vi "Teleop.vi"(10 "Match Info":T1={"Autonomous Elapsed Seconds"=0.0, "TeleOp Elapsed Seconds"=0.0, "Disabled Elapsed Seconds"=0.0, "Visited Autonomous"=FALSE, "Visited TeleOp"=FALSE, "Visited Disabled"=FALSE, "Autonomous Settings"={"Autonomous Style"=enum."Independent", "VI Refnum"=refnum}}, 11 "Call Context":T2) -> ()   [LabVIEW 2015]
doc: "This VI is called for each TeleOp packet received from the DS where the robot is not disabled. It is often used to read from the joysticks and update I/O or to update setpoints for timed control loops. It should complete and return within 20 milliseconds or it may miss DS packets."
uses:
  <vilib>/Rock Robotics/WPI/DriverStation/WPI_DriverStationDerivedRobotMode.ctl
  <vilib>/Rock Robotics/WPI/DriverStation/WPI_DriverStationMatch Info.ctl
  <vilib>/Rock Robotics/WPI/Solenoid/WPI_SolenoidValue.ctl
  <vilib>/Rock Robotics/WPI/Utilities/WPI_GetSetVariantRefNum.vi
  <vilib>/Rock Robotics/Network Tables/NT Write Boolean Array.vi
  <vilib>/Rock Robotics/Network Tables/NT Write Numeric Array.vi
  <vilib>/Rock Robotics/Network Tables/NT Read Boolean.vi
  <vilib>/Rock Robotics/Network Tables/NT Read Number.vi
  <vilib>/Rock Robotics/WPI/Solenoid/WPI_SolenoidSetEnum.vi
panel:
  out "Compressor Running":bool
  out "Enabled":bool
  out "Sample Slider 0":dbl(slide) scale=0.0..5.0
  out "Sample Boolean 1":bool
  out "Sample Boolean 0":bool
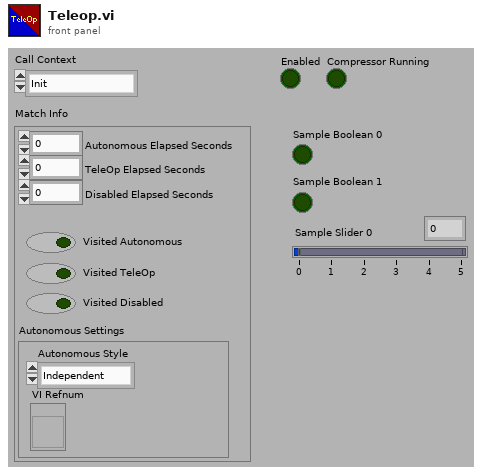
[diagram p1: front panel]
types:
  T1 = typedef "WPI_DriverStationMatch Info.ctl" = cluster{"Autonomous Elapsed Seconds":dbl, "TeleOp Elapsed Seconds":dbl, "Disabled Elapsed Seconds":dbl, "Visited Autonomous":bool, "Visited TeleOp":bool, "Visited Disabled":bool, "Autonomous Settings":cluster{"Autonomous Style":enum16{"Iterative", "Independent"}, "VI Refnum":refnum<vi>}}
  T2 = typedef "WPI_DriverStationDerivedRobotMode.ctl" = enum16{"Init", "Execute", "Stop"}
  T3 = typedef "WPI_SolenoidValue.ctl" = enum16{"Off", "On", "Forward", "Reverse"}
  T4 = typedef "WPI_RobotDriveDevRef.ctl" = cluster{"DevStatus":errorcluster, "Motors[]":T5[], "Square Inputs":bool, "Max Output":dbl}
  T5 = typedef "WPI_MotorControlDeviceRef.ctl" = cluster{"DeviceStatus":errorcluster, "Type":T6, "PWM":cluster{"PWM Channel":T7, "DeadBand":T8}, "CAN":cluster{"Device Number":u8, "Control Mode":T9, "Semaphore":T10, "Max Vout":dbl, "TalonSRX Control Mode":T11}, "Invert":bool}
  T6 = typedef "WPI_MotorControlType.ctl" = enum16{"PWM", "CAN", "CANTalonSRX"}
  T7 = typedef "FPGA_DIOPWMChannel.ctl" = enum8{"PWM 0", "PWM 1", "PWM 2", "PWM 3", "PWM 4", "PWM 5", "PWM 6", "PWM 7", "PWM 8", "PWM 9", "PWM MXP 0", "PWM MXP 1", "PWM MXP 2", "PWM MXP 3", "PWM MXP 4", "PWM MXP 5", "PWM MXP 6", "PWM MXP 7", "PWM MXP 8", "PWM MXP 9", "Invalid"}
  T8 = typedef "WPI_PWMDeadband.ctl" = cluster{"Name":string, "maxPositivePwm":i32, "minPositivePwm":i32, "centerPwm":i32, "maxNegativePwm":i32, "minNegativePwm":i32, "angularRange":u16}
  T9 = typedef "WPI_CANJaguar_ControlMode.ctl" = enum8{"Percent VBus", "Current", "Speed", "Position", "Voltage"}
  T10 = typedef "Semaphore RefNum" = refnum<k1>
  T11 = typedef "WPI_CANTalonSRX_APIControlMode.ctl" = enum8{"Percent VBus", "Speed", "Position", "Slave", "Unchanged / Invalid", "Voltage Compensation", "Current", "Motion Profile"}
  T12 = typedef "WPI_JoystickDevRef.ctl" = cluster{"Device":T13}
  T13 = typedef "WPI_JoystickDeviceEnum.ctl" = enum16{"USB 0", "USB 1", "USB 2", "USB 3", "USB 4", "USB 5"}
  T14 = typedef "WPI_CompressorDevRef.ctl" = cluster{"DevStatus":errorcluster, "Pneumatics Control Module":u8}
  T15 = typedef "WPI_DigitalInputDevRef.ctl" = cluster{"DevStatus":errorcluster, "DIO Channel":T16}
  T16 = typedef "FPGA_DIOChannel.ctl" = enum8{"DIO 0", "DIO 1", "DIO 2", "DIO 3", "DIO 4", "DIO 5", "DIO 6", "DIO 7", "DIO 8", "DIO 9", "DIO MXP 0", "DIO MXP 1", "DIO MXP 2", "DIO MXP 3", "DIO MXP 4", "DIO MXP 5", "DIO MXP 6", "DIO MXP 7", "DIO MXP 8", "DIO MXP 9", "DIO MXP 10", "DIO MXP 11", "DIO MXP 12", "DIO MXP 13", "DIO MXP 14", "DIO MXP 15", "Invalid"}
  T17 = typedef "WPI_SolenoidDevRef.ctl" = cluster{"DevStatus":errorcluster, "Pneumatics Control Module":u8, "Forward Solenoid Channel":T18, "Reverse Solenoid Channel":T18}
  T18 = typedef "WPI_SolenoidChannel.ctl" = enum8{"Solenoid 0", "Solenoid 1", "Solenoid 2", "Solenoid 3", "Solenoid 4", "Solenoid 5", "Solenoid 6", "Solenoid 7", "Invalid"}
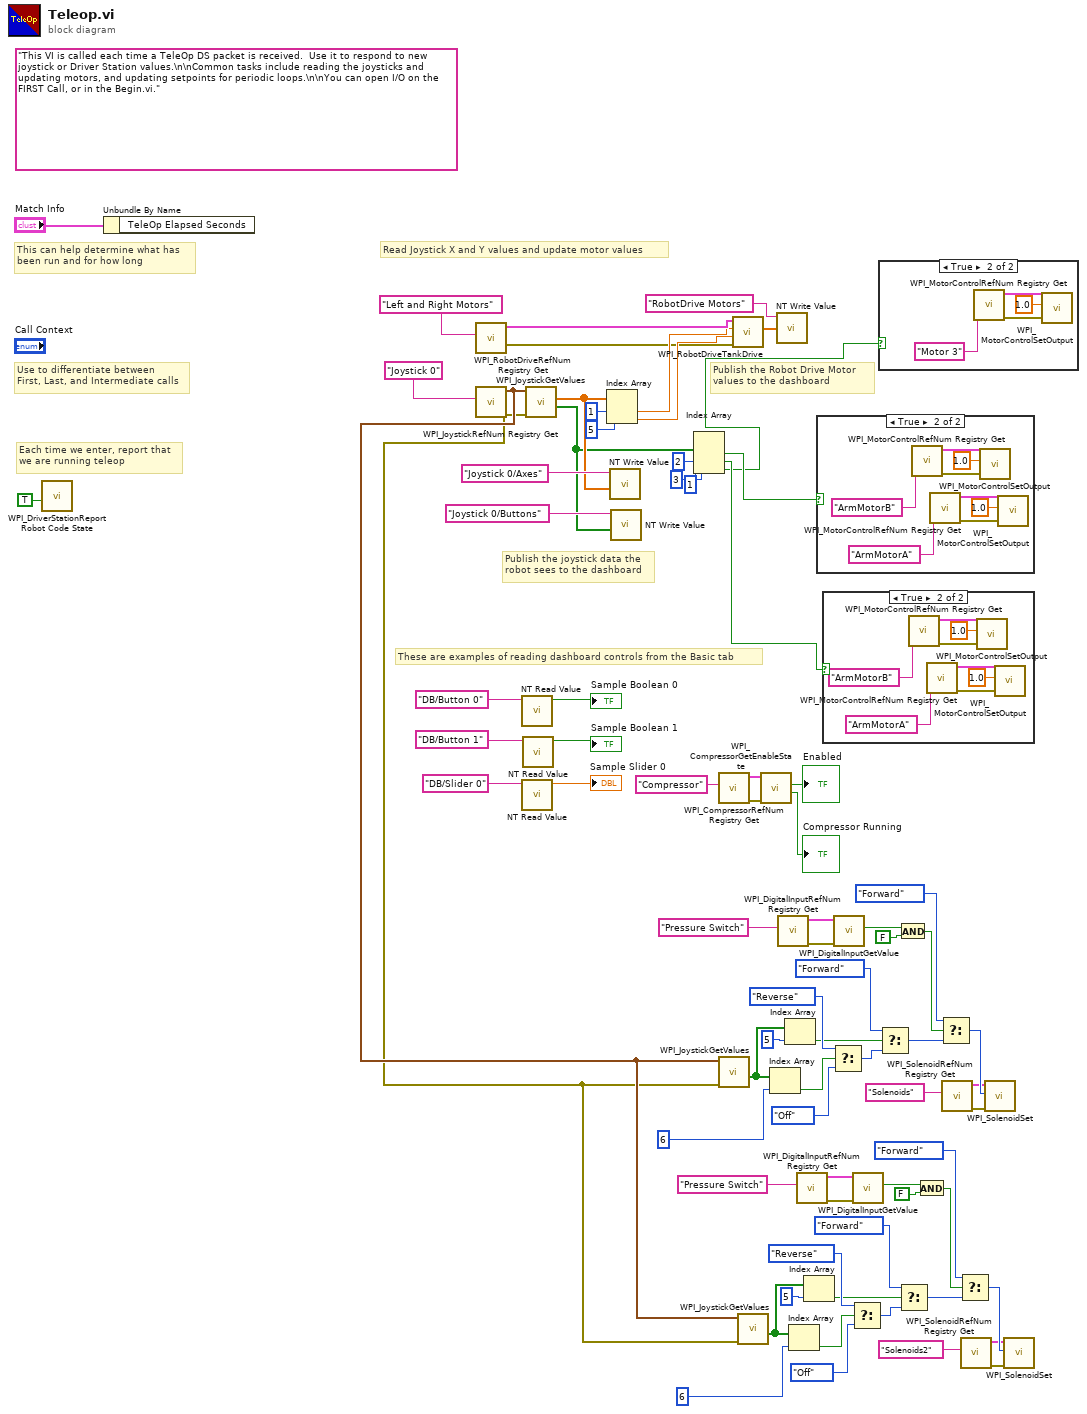
[diagram p0: block diagram]
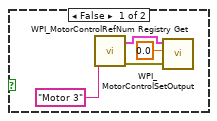
[diagram p2: hidden frame]
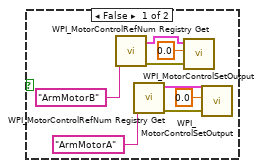
[diagram p3: hidden frame]
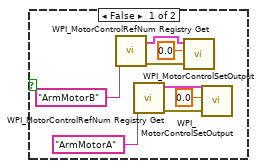
[diagram p4: hidden frame]
diagram:
  (unwired) "This VI is called each time a TeleOp DS packet is received.  Use it to respond to new joystick or Driver Station values.\n\nCommon tasks include reading the joysticks and updating motors, and updating setpoints for periodic loops.\n\nYou can open I/O on the FIRST Call, or in the Begin.vi."
  # "These are examples of reading dashboard controls from the Basic tab"
  # "Publish the Robot Drive Motor\nvalues to the dashboard"
  # "Publish the joystick data the\nrobot sees to the dashboard"
  # "Each time we enter, report that\nwe are running teleop"
  # "Use to differentiate between\nFirst, Last, and Intermediate calls"
  # "This can help determine what has\nbeen run and for how long"
  # "Read Joystick X and Y values and update motor values"
  n1 = call <vilib>:"WPI_DriverStationReport Robot Code State.vi"("TeleOp"=TRUE ("Autonomous")) -> ()  [unwired: 10 in, 1 out]
  n2 = Unbundle By Name("Match Info") -> ()  [unwired: 1 out]
  n3 = call <vilib>:"WPI_RobotDriveRefNum Registry Get.vi"("refnum name"="Left and Right Motors") -> ("error out"=w50:errorcluster, "RobotDriveDevRef"=w63:T4)  [unwired: 1 in, 8 out]
  n4 = call <vilib>:"WPI_JoystickRefNum Registry Get.vi"("refnum name"="Joystick 0") -> ("error out"=w1:errorcluster, "JoystickDevRef"=w2:T12)  [unwired: 1 in, 8 out]
  n5 = call-poly <vilib>:"NT Read Value.vi"("Name"="DB/Button 0" ("refnum name")) -> ("Boolean"=→"Sample Boolean 0":bool)  [unwired: 9 in, 1 out]
  n6 = call-poly <vilib>:"NT Read Value.vi"("Name"="DB/Slider 0" ("refnum name")) -> ("Numeric"=→"Sample Slider 0":dbl)  [unwired: 9 in, 1 out]
  n7 = call-poly <vilib>:"NT Read Value.vi"("Name"="DB/Button 1" ("refnum name")) -> ("Boolean"=→"Sample Boolean 1":bool)  [unwired: 9 in, 1 out]
  n8 = call <vilib>:"WPI_JoystickGetValues.vi"("error in (no error)"=w1, "JoystickDevRef"=w2) -> ("Buttons"=w57:bool[], "Axes"=w71:dbl[])  [unwired: 5 in, 3 out]
  n9 = Index Array(array=w71, index #1=1 ("index"), index #2=5 ("index")) -> (element #1=w62:dbl, element #2=w61:dbl)
  n10 = call-poly <vilib>:"NT Write Value.vi"("Numeric Array"=w71, "Name"="Joystick 0/Axes") -> ()  [unwired: 9 in, 1 out]
  n11 = call-poly <vilib>:"NT Write Value.vi"("Boolean Array"=w57, "Name"="Joystick 0/Buttons") -> ()  [unwired: 9 in, 1 out]
  n12 = Index Array(array=w57, index #1=1 ("index"), index #2=2 ("index"), index #3=3 ("index")) -> (element #1=w55:bool, element #2=w53:bool, element #3=w51:bool)
  n13 = call <vilib>:"WPI_CompressorRefNum Registry Get.vi"("refnum name"="Compressor") -> ("error out"=w47:errorcluster, "CompressorDevRef"=w48:T14)  [unwired: 9 in]
  n14 = call <vilib>:"WPI_JoystickGetValues.vi"("error in (no error)"=w1, "JoystickDevRef"=w2) -> ("Buttons"=w40:bool[])  [unwired: 5 in, 4 out]
  n15 = call <vilib>:"WPI_RobotDriveTankDrive.vi"("error in (no error)"=w50, "Right axis value"=w61, "Left axis value"=w62, "RobotDriveDevRef"=w63) -> ("Motor Values"=w58:dbl[])  [unwired: 5 in, 2 out]
  n16 = call <vilib>:"WPI_JoystickGetValues.vi"("error in (no error)"=w1, "JoystickDevRef"=w2) -> ("Buttons"=w19:bool[])  [unwired: 5 in, 4 out]
  n17 = call <vilib>:"WPI_CompressorGetEnableState.vi"("error in (no error)"=w47, "CompressorDevRef"=w48) -> ("Compressor Running"=→"Compressor Running":bool, "Enabled"=→"Enabled":bool)  [unwired: 6 in, 2 out]
  n18 = Index Array(array=w40, index=6) -> (element=w37:bool)
  n19 = call-poly <vilib>:"NT Write Value.vi"("Numeric Array"=w58, "Name"="RobotDrive Motors") -> ()  [unwired: 9 in, 1 out]
  n20 = call <vilib>:"WPI_DigitalInputRefNum Registry Get.vi"("refnum name"="Pressure Switch") -> ("error out"=w43:errorcluster, "DigitalInputDevRef"=w42:T15)  [unwired: 9 in]
  n21 = Index Array(array=w40, index=5) -> (element=w31:bool)
  n22 = Index Array(array=w19, index=6) -> (element=w16:bool)
  n23 = call <vilib>:"WPI_DigitalInputRefNum Registry Get.vi"("refnum name"="Pressure Switch") -> ("error out"=w22:errorcluster, "DigitalInputDevRef"=w21:T15)  [unwired: 9 in]
  n24 = Index Array(array=w19, index=5) -> (element=w10:bool)
  n25 = case shown="True" w55 {
    frame False {
      n26 = call <vilib>:"WPI_MotorControlRefNum Registry Get.vi"("refnum name"="ArmMotorB") -> ("error out"=w80:errorcluster, "MotorControlDevRef"=w78:T5)  [unwired: 9 in]
      n27 = call <vilib>:"WPI_MotorControlRefNum Registry Get.vi"("refnum name"="ArmMotorA") -> ("error out"=w83:errorcluster, "MotorControlDevRef"=w84:T5)  [unwired: 9 in]
      n28 = call <vilib>:"WPI_MotorControlSetOutput.vi"("error in (no error)"=w80, "Output"=0.0, "MotorControlDevRef"=w78) -> ()  [unwired: 6 in, 3 out]
      n29 = call <vilib>:"WPI_MotorControlSetOutput.vi"("error in (no error)"=w83, "Output"=0.0, "MotorControlDevRef"=w84) -> ()  [unwired: 6 in, 3 out]
    }
    frame True {
      n30 = call <vilib>:"WPI_MotorControlRefNum Registry Get.vi"("refnum name"="ArmMotorB") -> ("error out"=w87:errorcluster, "MotorControlDevRef"=w88:T5)  [unwired: 9 in]
      n31 = call <vilib>:"WPI_MotorControlRefNum Registry Get.vi"("refnum name"="ArmMotorA") -> ("error out"=w91:errorcluster, "MotorControlDevRef"=w92:T5)  [unwired: 9 in]
      n32 = call <vilib>:"WPI_MotorControlSetOutput.vi"("error in (no error)"=w87, "Output"=1.0, "MotorControlDevRef"=w88) -> ()  [unwired: 6 in, 3 out]
      n33 = call <vilib>:"WPI_MotorControlSetOutput.vi"("error in (no error)"=w91, "Output"=1.0, "MotorControlDevRef"=w92) -> ()  [unwired: 6 in, 3 out]
    }
  }
  n34 = case shown="True" w53 {
    frame False {
      n35 = call <vilib>:"WPI_MotorControlRefNum Registry Get.vi"("refnum name"="ArmMotorB") -> ("error out"=w96:errorcluster, "MotorControlDevRef"=w94:T5)  [unwired: 9 in]
      n36 = call <vilib>:"WPI_MotorControlRefNum Registry Get.vi"("refnum name"="ArmMotorA") -> ("error out"=w99:errorcluster, "MotorControlDevRef"=w100:T5)  [unwired: 9 in]
      n37 = call <vilib>:"WPI_MotorControlSetOutput.vi"("error in (no error)"=w96, "Output"=0.0, "MotorControlDevRef"=w94) -> ()  [unwired: 6 in, 3 out]
      n38 = call <vilib>:"WPI_MotorControlSetOutput.vi"("error in (no error)"=w99, "Output"=0.0, "MotorControlDevRef"=w100) -> ()  [unwired: 6 in, 3 out]
    }
    frame True {
      n39 = call <vilib>:"WPI_MotorControlRefNum Registry Get.vi"("refnum name"="ArmMotorB") -> ("error out"=w103:errorcluster, "MotorControlDevRef"=w104:T5)  [unwired: 9 in]
      n40 = call <vilib>:"WPI_MotorControlRefNum Registry Get.vi"("refnum name"="ArmMotorA") -> ("error out"=w107:errorcluster, "MotorControlDevRef"=w108:T5)  [unwired: 9 in]
      n41 = call <vilib>:"WPI_MotorControlSetOutput.vi"("error in (no error)"=w103, "Output"=1.0, "MotorControlDevRef"=w104) -> ()  [unwired: 6 in, 3 out]
      n42 = call <vilib>:"WPI_MotorControlSetOutput.vi"("error in (no error)"=w107, "Output"=1.0, "MotorControlDevRef"=w108) -> ()  [unwired: 6 in, 3 out]
    }
  }
  n43 = Select(t=WPI_SolenoidValue."Reverse" ("Value"), s=w37, f=WPI_SolenoidValue."Off" ("Value")) -> (s? t:f=w32:T3)
  n44 = call <vilib>:"WPI_DigitalInputGetValue.vi"("error in (no error)"=w43, "DigitalInputDevRef"=w42) -> ("Value"=w36:bool)  [unwired: 7 in, 2 out]
  n45 = Select(t=WPI_SolenoidValue."Reverse" ("Value"), s=w16, f=WPI_SolenoidValue."Off" ("Value")) -> (s? t:f=w11:T3)
  n46 = call <vilib>:"WPI_DigitalInputGetValue.vi"("error in (no error)"=w22, "DigitalInputDevRef"=w21) -> ("Value"=w15:bool)  [unwired: 7 in, 2 out]
  n47 = case shown="True" w51 {
    frame False {
      n48 = call <vilib>:"WPI_MotorControlRefNum Registry Get.vi"("refnum name"="Motor 3") -> ("error out"=w112:errorcluster, "MotorControlDevRef"=w110:T5)  [unwired: 9 in]
      n49 = call <vilib>:"WPI_MotorControlSetOutput.vi"("error in (no error)"=w112, "Output"=0.0, "MotorControlDevRef"=w110) -> ()  [unwired: 6 in, 3 out]
    }
    frame True {
      n50 = call <vilib>:"WPI_MotorControlRefNum Registry Get.vi"("refnum name"="Motor 3") -> ("error out"=w115:errorcluster, "MotorControlDevRef"=w116:T5)  [unwired: 9 in]
      n51 = call <vilib>:"WPI_MotorControlSetOutput.vi"("error in (no error)"=w115, "Output"=1.0, "MotorControlDevRef"=w116) -> ()  [unwired: 6 in, 3 out]
    }
  }
  n52 = Select(t=WPI_SolenoidValue."Forward" ("Value"), s=w31, f=w32) -> (s? t:f=w26:T3)
  n53 = And(x=w36, y=FALSE) -> (x .and. y?=w34:bool)
  n54 = Select(t=WPI_SolenoidValue."Forward" ("Value"), s=w10, f=w11) -> (s? t:f=w5:T3)
  n55 = And(x=w15, y=FALSE) -> (x .and. y?=w13:bool)
  n56 = Select(t=WPI_SolenoidValue."Forward" ("Value"), s=w34, f=w26) -> (s? t:f=w29:T3)
  n57 = call <vilib>:"WPI_SolenoidRefNum Registry Get.vi"("refnum name"="Solenoids") -> ("error out"=w27:errorcluster, "SolenoidDevRef"=w28:T17)  [unwired: 9 in]
  n58 = Select(t=WPI_SolenoidValue."Forward" ("Value"), s=w13, f=w5) -> (s? t:f=w8:T3)
  n59 = call <vilib>:"WPI_SolenoidRefNum Registry Get.vi"("refnum name"="Solenoids2") -> ("error out"=w6:errorcluster, "SolenoidDevRef"=w7:T17)  [unwired: 9 in]
  n60 = call-poly <vilib>:"WPI_SolenoidSet.vi"("error in (no error)"=w27, "Value"=w29, "SolenoidDevRef"=w28) -> ()  [unwired: 7 in, 2 out]
  n61 = call-poly <vilib>:"WPI_SolenoidSet.vi"("error in (no error)"=w6, "Value"=w8, "SolenoidDevRef"=w7) -> ()  [unwired: 7 in, 2 out]
